vi "Multi-Button State Selection.vi"() -> (0 "Selected State":string)   [LabVIEW 2019]
doc: "This VI is designed to convert (possibly conflicting) button presses (or other triggers) into a robot state string. While the triggers do not have to be instantaneous, you should design your human interfaces to never latch any state selection buttons. Disallowing states is also support. If a state is allowed after not previously being allowed, the state trigger must be reissued."
panel:
  in  "Issue 2":bool
  in  "Robot Tipping":bool
  out "Elevator Height (in)":dbl
  in  "State Names":string[](array[string])=["State A", "State B", "State C", "State D"]
  in  "State D":bool
  in  "State C":bool
  in  "State B":bool
  in  "State A":bool
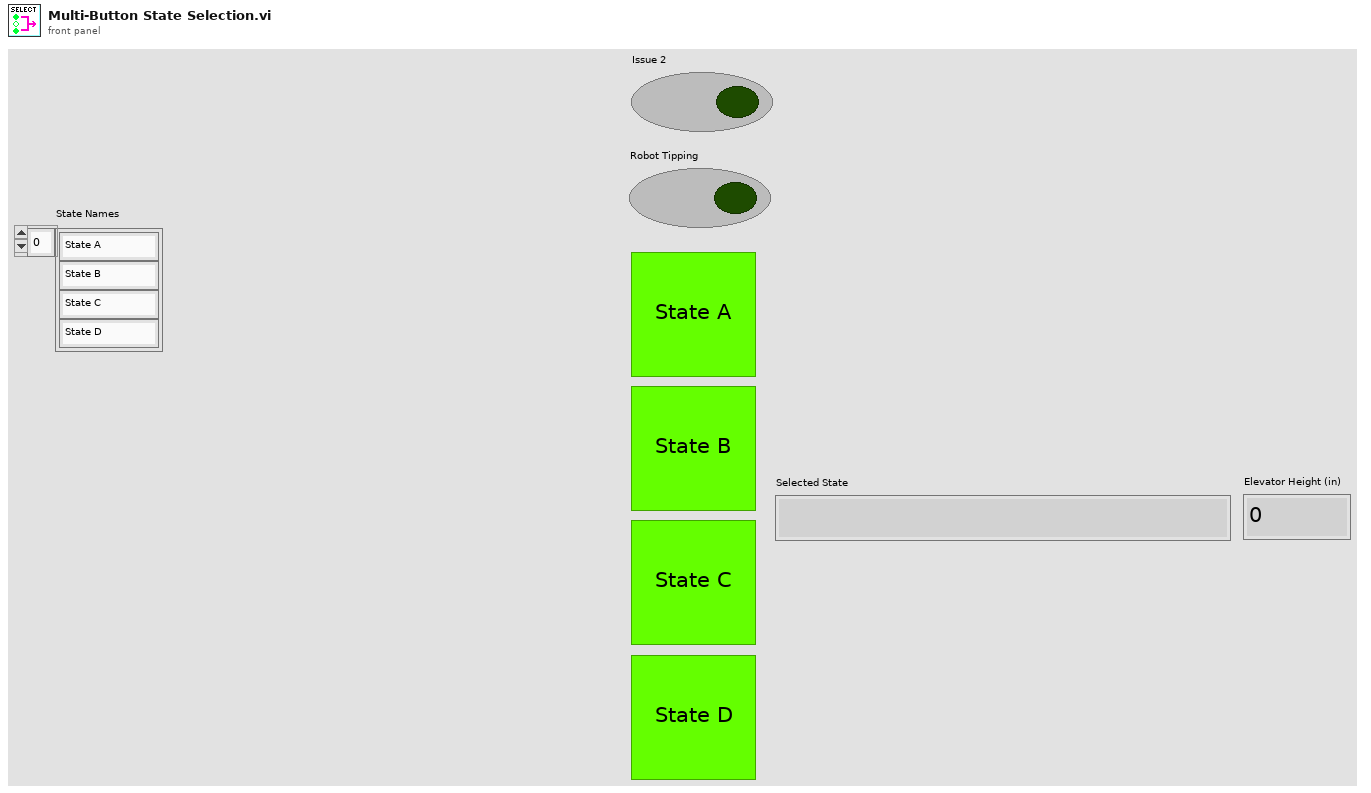
[diagram p1: front panel]
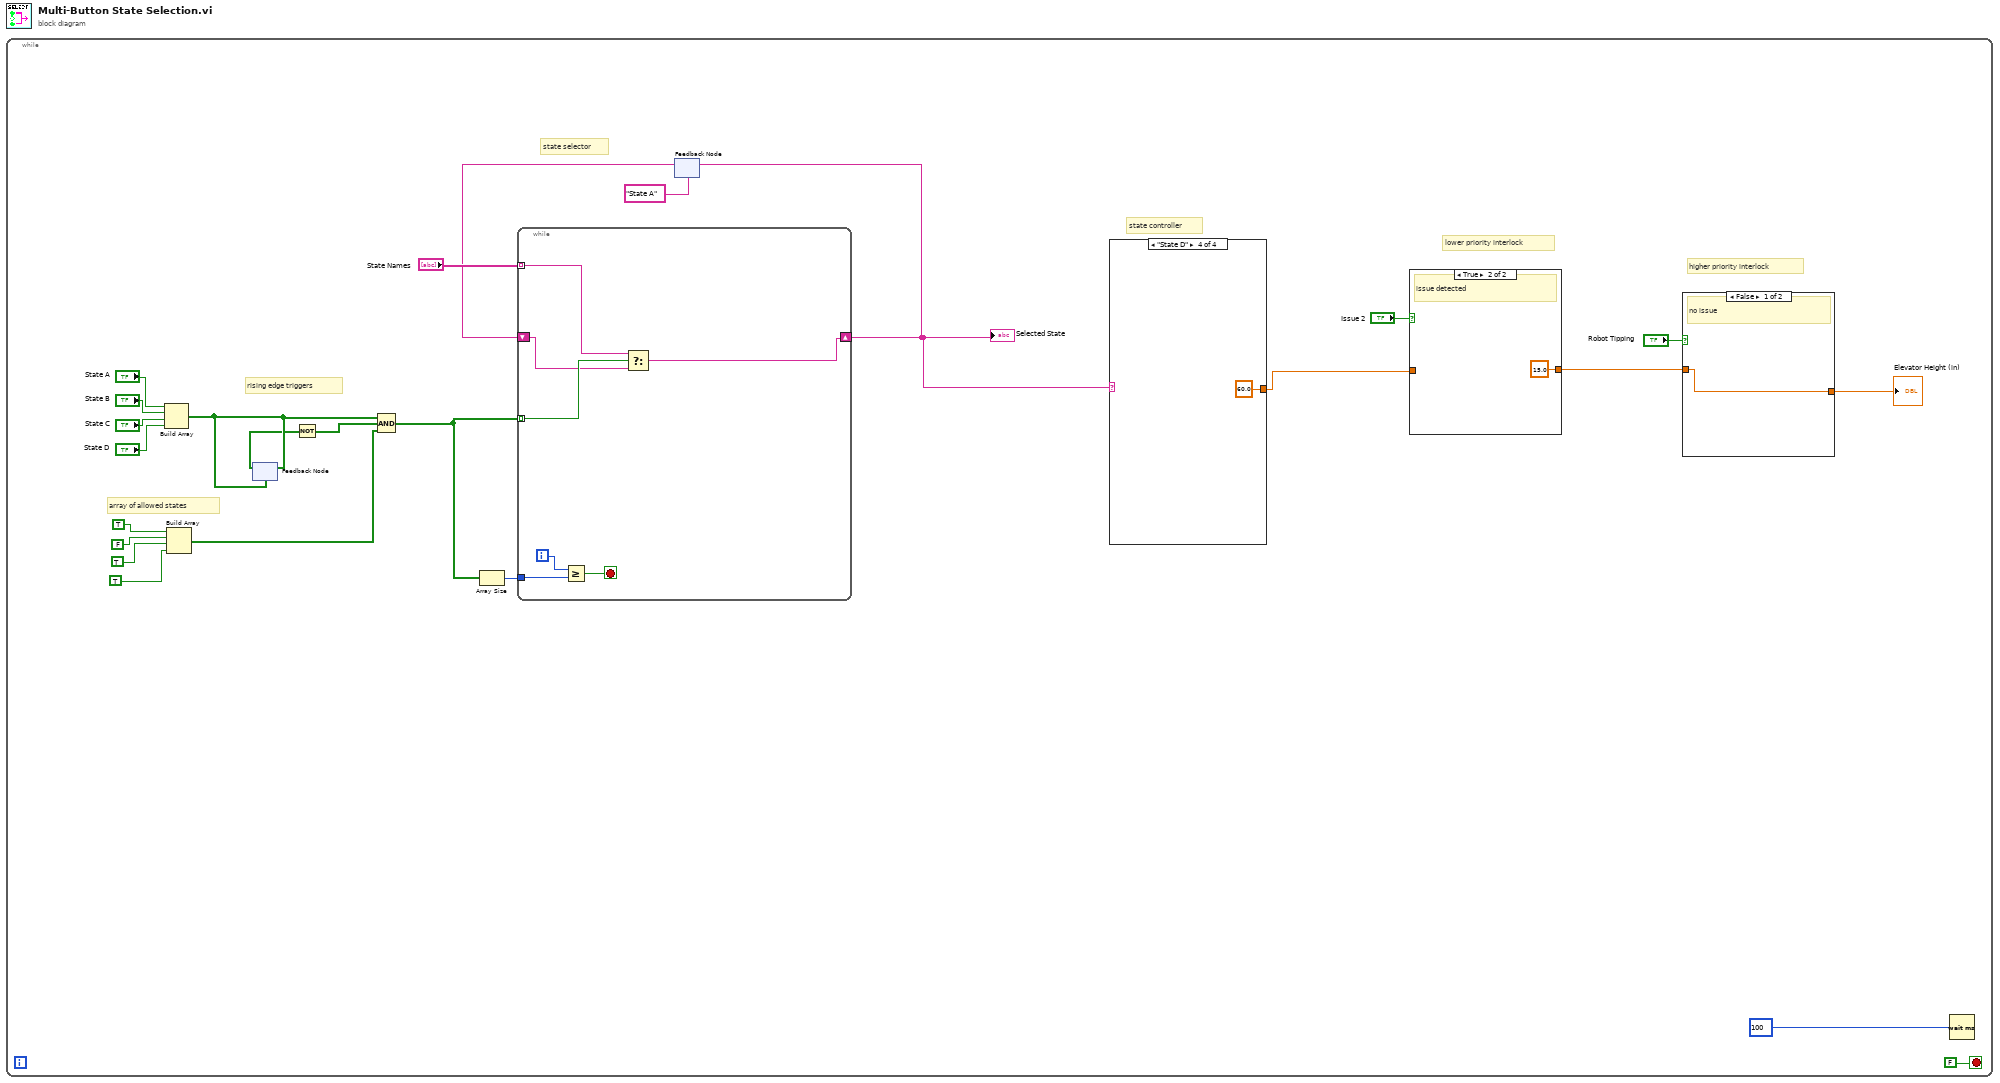
[diagram p0: block diagram]
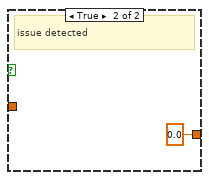
[diagram p3: hidden frame]
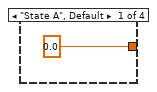
[diagram p4: hidden frame]
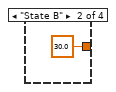
[diagram p5: hidden frame]
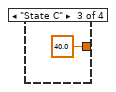
[diagram p6: hidden frame]
diagram:
  n1 = while {
    stop <- FALSE stop-if-true
    # "lower priority interlock"
    # "higher priority interlock"
    # "state selector"
    # "state controller"
    # "array of allowed states"
    # "rising edge triggers"
    n2 = Build Array("State A", "State B", "State C", "State D") -> (w19:bool[])
    n3 = Build Array(TRUE, FALSE, TRUE, TRUE) -> (w6:bool[])
    n4 = feedback-in #1(w19) -> ()
    n5 = feedback #1(w19) -> (w18:bool[])
    n6 = Not(x=w18) -> (.not. x?=w17:bool[])
    n7 = Compound Arithmetic op=AND(w19, w17, w6) -> (w16:bool[])
    n8 = Array Size(array=w16) -> (size(s)=w15:i32)
    n9 = feedback #2("State A") -> (w13:string)
    n10 = while {
      tunnel: w16 -> [w37] mode=indexing
      tunnel: w15 -> [w39]
      shift-right: [w35] -> w11
      shift-left: w13 -> [w36]
      tunnel: "State Names" -> [w34] mode=indexing
      i -> [w40]
      stop <- w38 stop-if-true
      n11 = Greater Or Equal?(x=w40, y=w39) -> (x >= y?=w38:bool)
      n12 = Select(t=w34, s=w37, f=w36) -> (s? t:f=w35:string)
    }
    "Selected State" <- w11
    n13 = feedback-in #2(w11) -> ()
    n14 = case shown="\"State D\"" w11 {
      tunnel: [0.0 30.0 40.0 60.0] -> w2
      frame "State A", Default {
      }
      frame "State B" {
      }
      frame "State C" {
      }
      frame "State D" {
      }
    }
    n15 = case shown="True" "Issue 2" {
      tunnel: [w26 15.0] -> w1
      tunnel: w2 -> [w26 _]
      frame False {
        # "no issue"
      }
      frame True {
        # "issue detected"
      }
    }
    n16 = case shown="False" "Robot Tipping" {
      tunnel: [w28 0.0] -> w5
      tunnel: w1 -> [w28 _]
      frame False {
        # "no issue"
      }
      frame True {
        # "issue detected"
      }
    }
    "Elevator Height (in)" <- w5
    n17 = Wait (ms)(milliseconds to wait=u32 100) -> ()  [unwired: 1 out]
  }
